vi "KepcoDCPwr Query Current Unit Protect Limit.vi"(0 "VISA Session":refnum<visa-resource-name>, 5 "Model In":string, 7 "channel name (\"\")":string="\"\"", 9 "Max Level (T),MIN LEVEL(F)":bool caption="Level", 11 "error in (no error)":errorcluster {"code" format="%.0x"}) -> (4 "VISA Session Out":refnum<visa-resource-name>, 6 "Model Out":string, 8 "channel name out (\"\")":string="\"\"" caption="channel name Out (\"\")", 10 "voltage level":dbl format="%^.2e", 15 "error out":errorcluster {"code" format="%.0x"})   [LabVIEW 2010]
doc: "This VI returns the maximum programmable voltage protect level that the power supply accepts. This limit may be configurable to find out unit limits use Volt Protect unit limit"
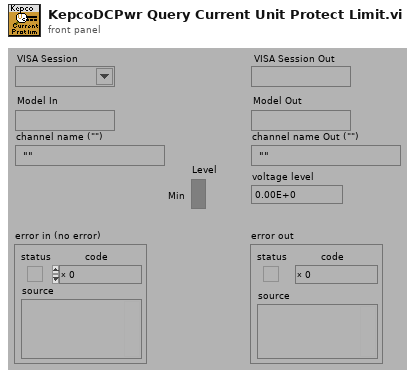
[diagram p1: front panel]
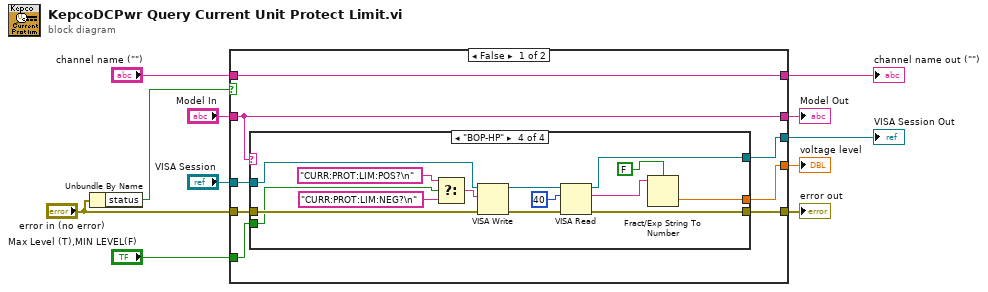
[diagram p0: block diagram]
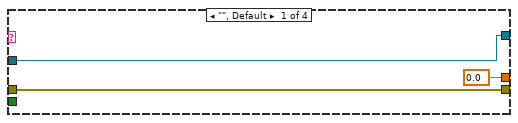
[diagram p2: hidden frame]
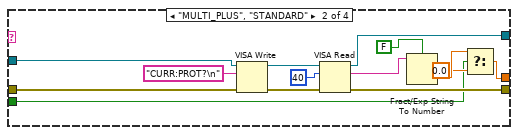
[diagram p3: hidden frame]
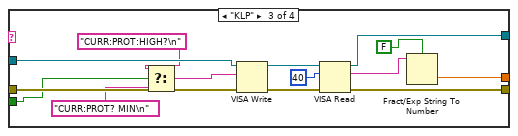
[diagram p4: hidden frame]
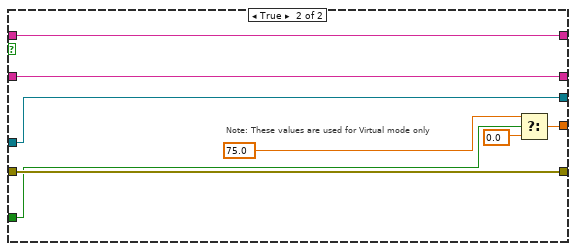
[diagram p5: hidden frame]
diagram:
  n1 = Unbundle By Name("error in (no error)") -> ("status"=w10:bool)
  n2 = case shown="False" w10 {
    tunnel: [w14 w72] -> w11
    tunnel: "error in (no error)" -> [w17 w72]
    tunnel: [w15 w71] -> w5
    tunnel: "VISA Session" -> [w18 w71]
    tunnel: [w16 w70] -> w4
    tunnel: "Model In" -> [w16 w70]
    tunnel: [w19 w69] -> w3
    tunnel: "channel name (\"\")" -> [w19 w69]
    tunnel: [w13 w66] -> w2
    tunnel: "Max Level (T),MIN LEVEL(F)" -> [w12 w68]
    frame False {
      n3 = case shown="\"BOP-HP\"" w16 {
        tunnel: w17 -> [w22 w36 w50 w64]
        tunnel: w18 -> [w20 w35 w49 w63]
        tunnel: [w20 w33 w47 w62] -> w15
        tunnel: [w22 w32 w46 w61] -> w14
        tunnel: [0.0 w25 w43 w59] -> w13
        tunnel: w12 -> [_ w23 w37 w57]
        frame "", Default {
        }
        frame "MULTI_PLUS", "STANDARD" {
          n4 = VISA Write(VISA resource name=w35, write buffer="CURR:PROT?\n", error in (no error)=w36) -> (VISA resource name out=w34:refnum<visa-resource-name>, error out=w31:errorcluster)  [unwired: 1 out]
          n5 = VISA Read(VISA resource name=w34, byte count=u32 40 ("byte count (0)"), error in (no error)=w31) -> (VISA resource name out=w33:refnum<visa-resource-name>, read buffer=w30:string, error out=w32:errorcluster)  [unwired: 1 out]
          n6 = Fract/Exp String To Number(use system decimal point (T)=FALSE, string=w30) -> (number=w26:dbl)  [unwired: 2 in, 1 out]
          n7 = Select(t=w26, s=w23, f=0.0) -> (s? t:f=w25:dbl)
        }
        frame "KLP" {
          n8 = Select(t="CURR:PROT:HIGH?\n", s=w37, f="CURR:PROT? MIN\n") -> (s? t:f=w39:string)
          n9 = VISA Write(VISA resource name=w49, write buffer=w39, error in (no error)=w50) -> (VISA resource name out=w48:refnum<visa-resource-name>, error out=w45:errorcluster)  [unwired: 1 out]
          n10 = VISA Read(VISA resource name=w48, byte count=u32 40 ("byte count (0)"), error in (no error)=w45) -> (VISA resource name out=w47:refnum<visa-resource-name>, read buffer=w44:string, error out=w46:errorcluster)  [unwired: 1 out]
          n11 = Fract/Exp String To Number(use system decimal point (T)=FALSE, string=w44) -> (number=w43:dbl)  [unwired: 2 in, 1 out]
        }
        frame "BOP-HP" {
          n12 = Select(t="CURR:PROT:LIM:POS?\n", s=w57, f="CURR:PROT:LIM:NEG?\n") -> (s? t:f=w54:string)
          n13 = VISA Write(VISA resource name=w63, write buffer=w54, error in (no error)=w64) -> (VISA resource name out=w52:refnum<visa-resource-name>, error out=w53:errorcluster)  [unwired: 1 out]
          n14 = VISA Read(VISA resource name=w52, byte count=u32 40 ("byte count (0)"), error in (no error)=w53) -> (VISA resource name out=w62:refnum<visa-resource-name>, read buffer=w60:string, error out=w61:errorcluster)  [unwired: 1 out]
          n15 = Fract/Exp String To Number(use system decimal point (T)=FALSE, string=w60) -> (number=w59:dbl)  [unwired: 2 in, 1 out]
        }
      }
    }
    frame True {
      # "Note: These values are used for Virtual mode only"
      n16 = Select(t=75.0, s=w68, f=0.0) -> (s? t:f=w66:dbl)
    }
  }
  "error out" <- w11
  "channel name out (\"\")" <- w3
  "Model Out" <- w4
  "VISA Session Out" <- w5
  "voltage level" <- w2
